vi "initStim.vi"(5 "ITA channel":dbl, 6 "ITI":dbl, 7 "Pulse Duration":dbl, 8 "error in (no error)":errorcluster, 9 "semicolon seperated stimuli":string, 10 "Lines":string[](array[string])=["Dev3/port0/line0", "Dev3/port0/line1", "Dev3/port0/line2", "Dev3/port0/line3", "Dev3/port0/line4"], 11 "Stim in":refnum<class "Stim.lvclass">) -> (0 "error out":errorcluster, 3 "Stim out":refnum<class "Stim.lvclass">)   [LabVIEW 2014, in "Stim.lvclass"]
uses:
  Stim.lvclass
  Stim.lvclass/Stim.ctl
  <vilib>/DAQmx/create/channels.llb/DAQmx Create Channel (DO-Digital Output).vi
  <resource>/objmgr/daqmx.rc
panel:
  in  "Stim Queue":T1
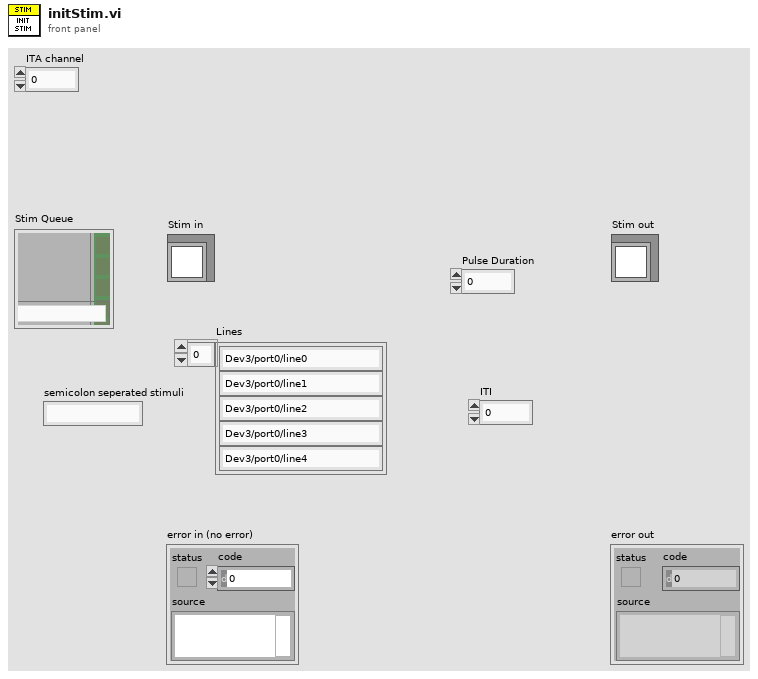
[diagram p1: front panel]
types:
  T1 = cluster{"Stimulus channels":bool[], "Stimulus":string}
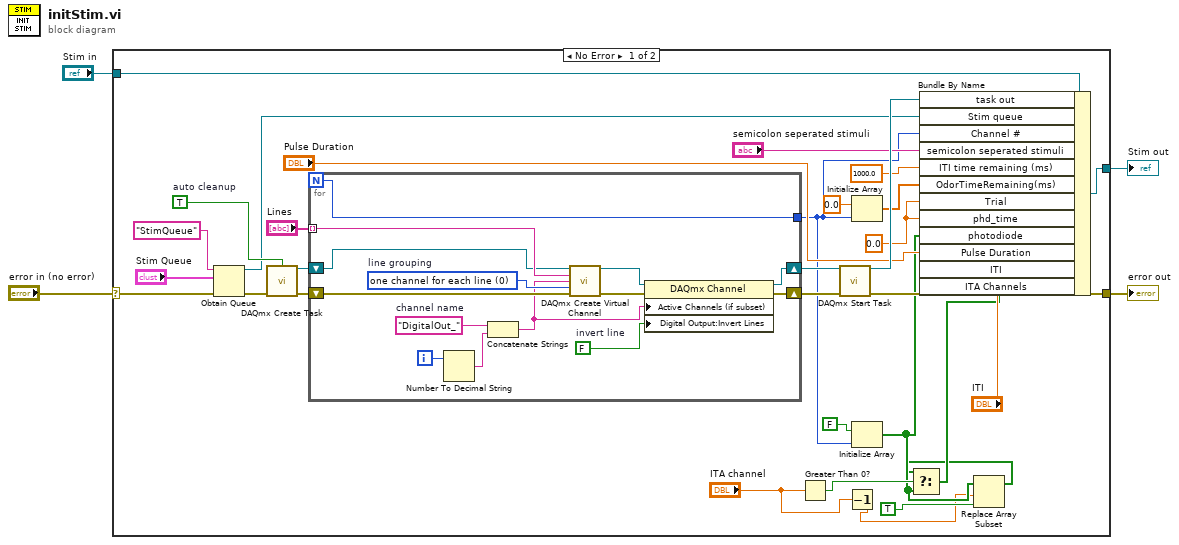
[diagram p0: block diagram]
diagram:
  n1 = case shown="No Error" "error in (no error)" {
    selector: "error in (no error)" -> [w26 w51]
    tunnel: [w31 w51] -> w1
    tunnel: [w34 w50] -> w2
    tunnel: "Stim in" -> [w35 w50]
    frame No Error {
      w15 = 0.0 ("Trial")
      w33 = TRUE  # auto cleanup
      n2 = Obtain Queue(name (unnamed)="StimQueue", element data type="Stim Queue", error in (no error)=w26) -> (queue out=w21:refnum<queue>, error out=w23:errorcluster)  [unwired: 2 in, 1 out]
      n3 = call <vilib>:"DAQmx Create Task.vi"("auto cleanup"=w33, "error in"=w23) -> ("task out"=w29:refnum<k21>, "error out"=w28:errorcluster)  [unwired: 12 in]
      n4 = for {
        N -> [w36]
        tunnel: "Lines" -> [w45] mode=indexing
        shift-right: [w39] -> w25
        shift-left: w29 -> [w44]
        shift-right: [w38] -> w24
        shift-left: w28 -> [w42]
        tunnel: [w36] -> w12
        i -> [w46]
        w43 = 0 items=["one channel for each line", "one channel for all lines"]  # line grouping
        w48 = "DigitalOut_"  # channel name
        w49 = FALSE  # invert line
        n5 = Number To Decimal String(number=w46) -> (decimal integer string=w47:string)  [unwired: 1 in]
        n6 = Concatenate Strings(w48, w47) -> (w37:string)
        n7 = call-poly <vilib>:"DAQmx Create Virtual Channel.vi"("task in"=w44, "lines"=w45, "name to assign"=w37, "line grouping"=w43, "error in"=w42) -> ("task out"=w40:refnum<k21>, "error out"=w41:errorcluster)  [unwired: 9 in]
        n8 = property class="DAQmx Channel"(reference=w40, error in=w41, "Active Channels (if subset)"=w37, "Digital Output:Invert Lines"=w49) -> (reference out=w39:refnum<k21>, error out=w38:errorcluster)
      }
      n9 = Greater Than 0?(x="ITA channel") -> (x > 0?=w11:bool)
      n10 = call <vilib>:"DAQmx Start Task.vi"("task/channels in"=w25, "error in"=w24) -> ("task out"=w32:refnum<k21>, "error out"=w31:errorcluster)  [unwired: 12 in]
      n11 = Decrement(x="ITA channel") -> (x-1=w6:dbl)
      n12 = Initialize Array(0.0 ("element"), w12) -> (w18:dbl[])
      n13 = Initialize Array(FALSE, w12) -> (w9:bool[])
      n14 = Replace Array Subset(array=w9, new element=TRUE, index=w6) -> (w5:bool[])
      n15 = Select(t=w5, s=w11, f=w9) -> (s? t:f=w10:bool[])
      n16 = Bundle By Name(cluster=w35, "task out"=w32, "Stim queue"=w21, "Channel #"=w12, "semicolon seperated stimuli"="semicolon seperated stimuli", "ITI time remaining (ms)"=1000.0, "OdorTimeRemaining(ms)"=w18, "Trial"=w15, "phd_time"=w15, "photodiode"=w9, "Pulse Duration"="Pulse Duration", "ITI"="ITI", "ITA Channels"=w10) -> (w34:refnum<class "Stim.lvclass">)
    }
    frame Error {
    }
  }
  "error out" <- w1
  "Stim out" <- w2
